vi "DFD Plot Freq Response (Log-Spaced).vi"(5 "output option":u16(ring) items=["Auto", "Floating-Point Only", "Fixed-Point Only"], 6 "fs [Hz]":dbl=-1.0 format="%.2f", 7 "plot settings":T1={"# freq bins"=-1, "low frequency [Hz]"=-1.0, "high frequency [Hz]"=-1.0}, 8 "error in (no error)":errorcluster, 9 "dB on? (T)":bool=TRUE, 10 "phase view":T8, 11 "filter in":T2={"mSRate_Fs"=1.0, "mSRate_Version"="2.0", "mSRate_Comments"="", "mSRate_OrgCoef"={"type"=enum."Undefined", "gain"=1.0, "coef a (k)"=[], "coef b (v)"=[]}, "mSRate_CurCoef"={"type"=enum."Undefined", "gain"=1.0, "coef a (k)"=[], "coef b (v)"=[]}, "mSRate_Quantized?"=FALSE, "mSRate_QCoef"={"type"=enum."Undefined", "gain"=1.0, "coef a (k)"=[], "coef b (v)"=[]}, "mSRate_QSettings"=[], "mSRate_Order"=0, "mSRate_Scaling"={"mSRate_ScaleByPowerOf2?"=FALSE, "mSRate_ScaleType"=enum."No Norm"}} {"mSRate_QSettings"."source" items=["Coef a/k"=0, "Coef b/v"=7, "Input"=1, "Output"=2, "Multiplicand"=3, "Product"=4, "Sum"=5, "Delay"=6, "Gain"=8]}) -> (0 "error out":errorcluster, 1 "phase response":cluster{"bins":dbl[], "response FXP":dbl[]}[](graph), 2 "magnitude response":cluster{"bins":dbl[], "response FXP":dbl[]}[](graph), 3 "filter out":T2={"mSRate_Fs"=1.0, "mSRate_Version"="2.0", "mSRate_Comments"="", "mSRate_OrgCoef"={"type"=enum."Undefined", "gain"=1.0, "coef a (k)"=[], "coef b (v)"=[]}, "mSRate_CurCoef"={"type"=enum."Undefined", "gain"=1.0, "coef a (k)"=[], "coef b (v)"=[]}, "mSRate_Quantized?"=FALSE, "mSRate_QCoef"={"type"=enum."Undefined", "gain"=1.0, "coef a (k)"=[], "coef b (v)"=[]}, "mSRate_QSettings"=[], "mSRate_Order"=0, "mSRate_Scaling"={"mSRate_ScaleByPowerOf2?"=FALSE, "mSRate_ScaleType"=enum."No Norm"}} {"mSRate_QSettings"."source" items=["Coef a/k"=0, "Coef b/v"=7, "Input"=1, "Output"=2, "Multiplicand"=3, "Product"=4, "Sum"=5, "Delay"=6, "Gain"=8]})   [LabVIEW 2017, in "NI_DigFilterLicensed.lvlib"]
doc: "Plots the frequency responses, including the magnitude and phase responses, of a filter."
uses:
  <vilib>/addons/Digital Filter Design/NI_DigFilterLicensed.lvlib
  <vilib>/addons/Digital Filter Design/_Objects.llb/DFD Filter Obj.ctl
  <vilib>/addons/Digital Filter Design/_Objects.llb/DFD Filter Coef.ctl
  <vilib>/addons/Digital Filter Design/_Objects.llb/DFD Filter Structure Type Selector.ctl
  <vilib>/addons/Digital Filter Design/_Objects.llb/dfd_Internal Quantization Settings.ctl
  <vilib>/addons/Digital Filter Design/_Objects.llb/dfd_Internal Quantization Srcs.ctl
  <vilib>/addons/Digital Filter Design/_Objects.llb/DFD Coef Norm Type.ctl
  <vilib>/addons/Digital Filter Design/_Objects.llb/DFD Phase Setting.ctl
  <vilib>/addons/Digital Filter Design/_Objects.llb/DFD Plot Settings.ctl
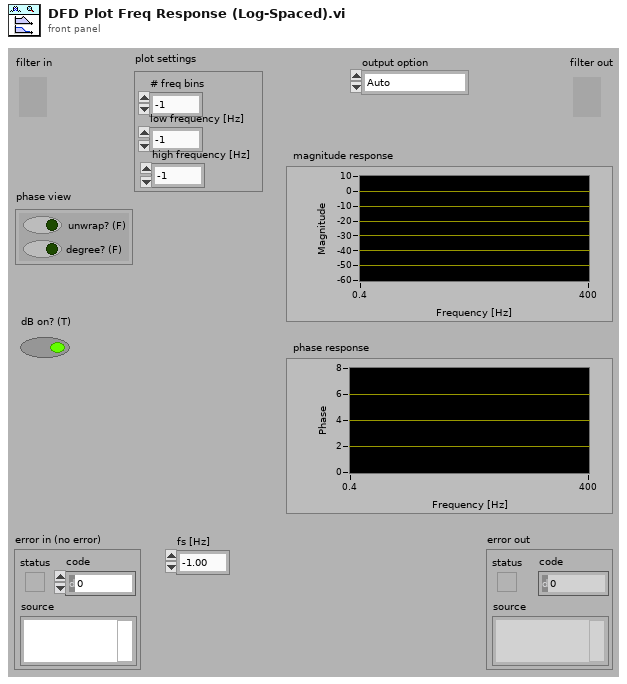
[diagram p1: front panel]
types:
  T1 = typedef "NI_DigFilterLicensed.lvlib/DFD Plot Settings.ctl" = cluster{"# freq bins":i32, "low frequency [Hz]":dbl, "high frequency [Hz]":dbl}
  T2 = typedef "NI_DigFilterLicensed.lvlib/DFD Filter Obj.ctl" = cluster{"mSRate_Fs":dbl, "mSRate_Version":string, "mSRate_Comments":string, "mSRate_OrgCoef":T3, "mSRate_CurCoef":T3, "mSRate_Quantized?":bool, "mSRate_QCoef":T3, "mSRate_QSettings":T5[], "mSRate_Order":i32, "mSRate_Scaling":cluster{"mSRate_ScaleByPowerOf2?":bool, "mSRate_ScaleType":T7}}
  T3 = typedef "NI_DigFilterLicensed.lvlib/DFD Filter Coef.ctl" = cluster{"type":T4, "gain":dbl, "coef a (k)":dbl[], "coef b (v)":dbl[]}
  T4 = typedef "NI_DigFilterLicensed.lvlib/DFD Filter Structure Type Selector.ctl" = enum16{"Undefined", "FIR Direct Form", "FIR Direct Form Transposed", "FIR Symmetric", "FIR Antisymmetric", "IIR Direct Form I", "IIR Direct Form I Transposed", "IIR Direct Form II", "IIR Direct Form II Transposed", "IIR Cascaded Second Order Sections Form I", "IIR Cascaded Second Order Sections Form I Transposed", "IIR Cascaded Second Order Sections Form II", "IIR Cascaded Second Order Sections Form II Transposed", "Lattice Allpass (basic sections)", "Lattice Allpass (one multiplier sections)", "Lattice Allpass (normalized sections)", "Lattice AR (basic sections)", "Lattice AR (one multiplier sections)", "Lattice AR (normalized sections)", "Lattice MA (minimum phase)", "Lattice MA (maximum phase)", "Lattice ARMA (basic sections)", "Lattice ARMA (one multiplier sections)", "Lattice ARMA (normalized sections)"}
  T5 = typedef "NI_DigFilterLicensed.lvlib/dfd_Internal Quantization Settings.ctl" = cluster{"source":T6, "wl":i16, "iwl":i16, "overflow mode":enum16{"Saturation", "Wrap"}, "rounding mode":enum16{"Nearest", "Truncation"}, "signed?":bool}
  T6 = typedef "NI_DigFilterLicensed.lvlib/dfd_Internal Quantization Srcs.ctl" = u16
  T7 = typedef "NI_DigFilterLicensed.lvlib/DFD Coef Norm Type.ctl" = enum16{"No Norm", "Time Domain 1-Norm", "Time Domain 2-Norm", "Time Domain Inf-Norm"}
  T8 = typedef "NI_DigFilterLicensed.lvlib/DFD Phase Setting.ctl" = cluster{"unwrap? (F)":bool, "degree? (F)":bool}
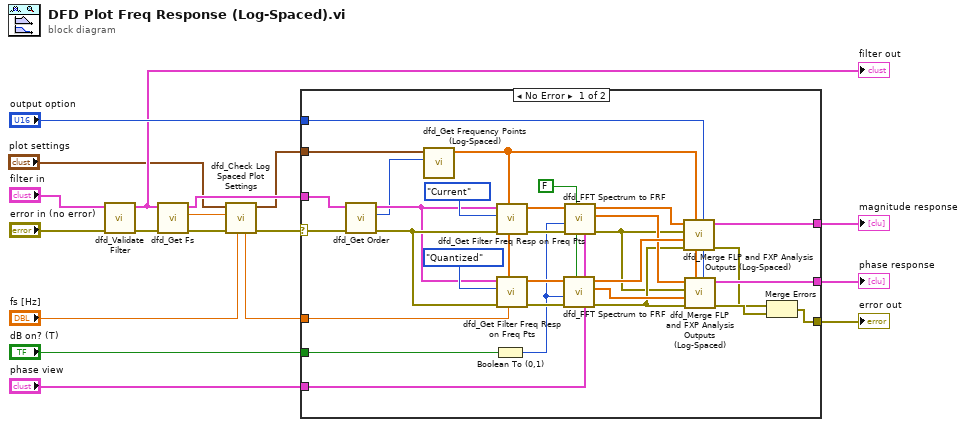
[diagram p0: block diagram]
diagram:
  n1 = call <vilib>:"dfd_Validate Filter.vi"("error in (no error)"="error in (no error)", "filter in"="filter in") -> ("error out"=w11:errorcluster, "filter out"=w12:T2)  [unwired: 1 in, 7 out]
  "filter out" <- w12
  n2 = call <vilib>:"dfd_Get Fs.vi"("error in (no error)"=w11, "filter in"=w12) -> ("error out"=w9:errorcluster, "fs [Hz]"=w1:dbl, "filter out"=w10:T2)  [unwired: 7 out]
  n3 = call <vilib>:"dfd_Check Log Spaced Plot Settings.vi"("fs [Hz] in"="fs [Hz]", "error in (no error)"=w9, "filter fs[Hz]"=w1, "plot settings"="plot settings") -> ("error out"=w8:errorcluster, "plot settings out"=w6:T1, "fs out [Hz]"=w4:dbl)  [unwired: 5 in]
  n4 = case shown="No Error" w8 {
    selector: w8 -> [w24 w49]
    tunnel: "phase view" -> [w36 _]
    tunnel: "dB on? (T)" -> [w45 _]
    tunnel: w4 -> [w20 _]
    tunnel: [w47 w49] -> w16
    tunnel: "output option" -> [w27 _]
    tunnel: [w46 _] -> w2
    tunnel: w6 -> [w25 _]
    tunnel: [w33 _] -> w3
    tunnel: w10 -> [w22 _]
    frame No Error {
      w40 = FALSE ("use half band?")
      n5 = call <vilib>:"dfd_Get Order.vi"("error in (no error)"=w24, "filter in"=w22) -> ("error out"=w23:errorcluster, "order"=w19:i32, "filter out"=w21:T2)  [unwired: 7 out]
      n6 = call <vilib>:"dfd_Get Frequency Points (Log-Spaced).vi"("order"=w19, "plot settings"=w25) -> ("freq points"=w26:dbl[])  [unwired: 9 in]
      n7 = Boolean To (0,1)(Boolean=w45) -> (0, 1=w37:i16)
      n8 = call <vilib>:"dfd_Get Filter Freq Resp on Freq Pts.vi"("fs [Hz]"=w20, "freqs [Hz]"=w26, "error in (no error)"=w23, "coef source"=enum16{"Original", "Current", "Quantized"}."Current", "filter in"=w21) -> ("error out"=w42:errorcluster, "freq response"=w43:cdb[])  [unwired: 3 in, 2 out]
      n9 = call <vilib>:"dfd_Get Filter Freq Resp on Freq Pts.vi"("fs [Hz]"=w20, "freqs [Hz]"=w26, "error in (no error)"=w23, "coef source"=enum16{"Original", "Current", "Quantized"}."Quantized", "filter in"=w21) -> ("error out"=w38:errorcluster, "freq response"=w39:cdb[])  [unwired: 3 in, 2 out]
      n10 = call <vilib>:"dfd_FFT Spectrum to FRF.vi"("phase view"=w36, "use half band?"=w40, "error in (no error)"=w38, "magnitude"=w37, "FFT {X}"=w39) -> ("error out"=w30:errorcluster, "phase"=w31:dbl[], "amplitude"=w34:dbl[])  [unwired: 1 in, 3 out]
      n11 = call <vilib>:"dfd_FFT Spectrum to FRF.vi"("phase view"=w36, "use half band?"=w40, "error in (no error)"=w42, "magnitude"=w37, "FFT {X}"=w43) -> ("error out"=w29:errorcluster, "phase"=w32:dbl[], "amplitude"=w35:dbl[])  [unwired: 1 in, 3 out]
      n12 = call <vilib>:"dfd_Merge FLP and FXP Analysis Outputs (Log-Spaced).vi"("output option"=w27, "frequency points"=w26, "error in FXP"=w30, "response FXP"=w34, "error in FLP"=w29, "response FLP"=w35) -> ("error out"=w28:errorcluster, "freq responses"=w33:cluster{"bins":dbl[], "response FXP":dbl[]}[])  [unwired: 4 in]
      n13 = call <vilib>:"dfd_Merge FLP and FXP Analysis Outputs (Log-Spaced).vi"("output option"=w27, "frequency points"=w26, "error in FXP"=w30, "response FXP"=w31, "error in FLP"=w29, "response FLP"=w32) -> ("error out"=w48:errorcluster, "freq responses"=w46:cluster{"bins":dbl[], "response FXP":dbl[]}[])  [unwired: 4 in]
      n14 = Merge Errors(w28, w48) -> (w47:errorcluster)
    }
    frame Error {
    }
  }
  "error out" <- w16
  "magnitude response" <- w3
  "phase response" <- w2
